vi "dfd_DFXP negate (ss).vi"(9 "High 64":i64 format="%.0x", 10 "Low 64":u64 format="%.0x") -> (1 "High 64":i64 format="%.0x", 2 "Low 64":u64 format="%.0x")   [LabVIEW 2017, in "NI_DigFilter_FXP.lvlib"]
uses:
  <vilib>/addons/Digital Filter Design/NI_DigFilter_FXP.lvlib
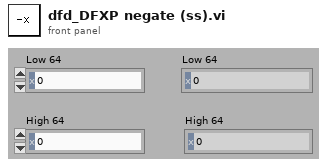
[diagram p1: front panel]
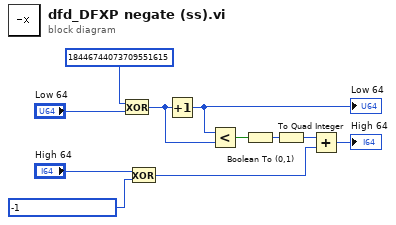
[diagram p0: block diagram]
diagram:
  n1 = Exclusive Or(1:"Low 64", 2:u64 18446744073709551615 ("y")) -> (0:w1:u64)
  n2 = Exclusive Or(1:i64 -1 ("y"), 2:"High 64") -> (0:w4:i64)
  n3 = Increment(x=w1) -> (x+1=w7:u64)
  "Low 64" <- w7
  n4 = Less?(x=w7, y=w1) -> (x < y?=w6:bool)
  n5 = Boolean To (0,1)(Boolean=w6) -> (0, 1=w5:i16)
  n6 = To Quad Integer(1:w5) -> (0:w3:i64)
  n7 = Add(x=w3, y=w4) -> (x+y=→"High 64":i64)
